vi "Hypergeometric CDF.vi"(8 "n":i32=20, 9 "k":i32=30, 10 "M":i32=100, 11 "x":dbl=4.0) -> (0 "error":i32, 3 "cdf(x)":dbl=0.2091632008258143)   [LabVIEW 2017, in "NI_Gmath.lvlib"]
doc: "Computes the discrete cumulative distribution function (CDF), or the probability that the random variate X, where X describes the selected distribution type, takes on a value less than or equal to <B>x</B>. You must manually select the polymorphic instance to use."
uses:
  <vilib>/gmath/NI_Gmath.lvlib
panel:
  # "Hypergeometric CDF"
  # "size of population"
  # "items"
  # "samples drawn"
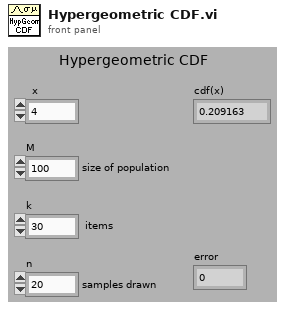
[diagram p1: front panel]
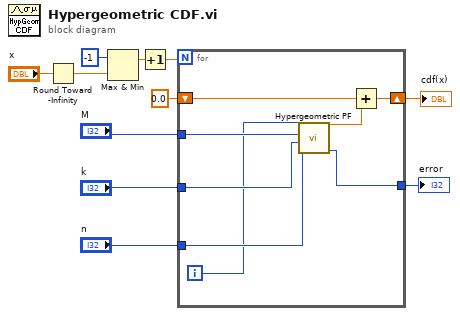
[diagram p0: block diagram]
diagram:
  n1 = Round Toward -Infinity(1:"x") -> (0:w1:dbl)
  n2 = Max & Min(x=-1, y=w1) -> (max(x,y)=w5:dbl)  [unwired: 1 out]
  n3 = Increment(x=w5) -> (x+1=w8:dbl)
  n4 = for {
    N: w8 -> [_]
    tunnel: [w19] -> w11
    tunnel: "M" -> [w18]
    tunnel: "k" -> [w17]
    tunnel: "n" -> [w16]
    shift-right: [w14] -> w7
    shift-left: 0.0 -> [w13]
    i -> [w15]
    n5 = call <vilib>:"Hypergeometric PF.vi"("n"=w16, "k"=w17, "M"=w18, "x"=w15) -> ("error"=w19:i32, "prob(x)"=w12:dbl)  [unwired: 6 in]
    n6 = Add(x=w13, y=w12) -> (x+y=w14:dbl)
  }
  "cdf(x)" <- w7
  "error" <- w11
